vi "Read Waveform.vi"(6 "wait for reply (T)":bool=TRUE, 8 "error in":errorcluster, 10 "Parameters 3":T1, 11 "Module ID":i32=-1) -> (0 "error out":errorcluster, 1 "timed out?":bool)   [LabVIEW 2020, in "Osciloscope Tektronix.lvlib"]
doc: "_____\nCreated using DQMH Event Scripter 6.0.0.122."
uses:
  Osciloscope Tektronix.lvlib
  Read Waveform Argument--cluster.ctl
  Read Waveform (Reply Payload)--cluster.ctl
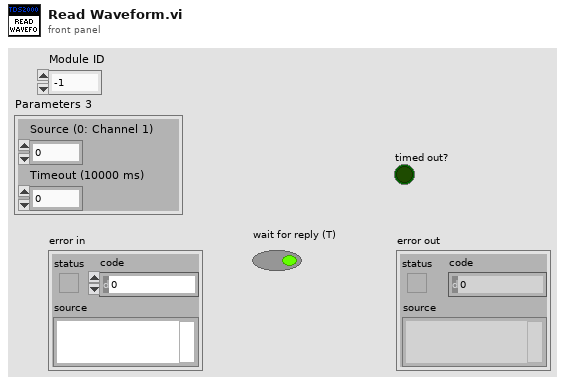
[diagram p1: front panel]
types:
  T1 = cluster{"Source (0: Channel 1)":u16, "Timeout (10000 ms)":u32}
  T2 = typedef "Osciloscope Tektronix.lvlib/Read Waveform Argument--cluster.ctl" = cluster{"Module ID":i32, "Wait Notifier":refnum<notifier>, "wait for reply":bool, "Parameters 3":cluster{"Source (0: Channel 1)":u16, "Timeout (10000 ms)":u32}}
  T3 = typedef "Osciloscope Tektronix.lvlib/Request Events--cluster.ctl" = cluster{"Stop Module":refnum<user-event>, "Show Panel":refnum<user-event>, "Hide Panel":refnum<user-event>, "Show Diagram":refnum<user-event>, "Get Module Execution Status":refnum<user-event>, "SET COM Port":refnum<user-event>, "Initialize Oscilloscope":refnum<user-event>, "Close Oscilloscope":refnum<user-event>, "AutoSetup":refnum<user-event>, "Configure Channel":refnum<user-event>, "Reset":refnum<user-event>, "Read Waveform":refnum<user-event>, "Read Measurement":refnum<user-event>, "Read Measurement 2 channels":refnum<user-event>}
  T4 = typedef "Osciloscope Tektronix.lvlib/Read Waveform (Reply Payload)--cluster.ctl" = cluster{"Read Waveform_error":errorcluster, "Waveform Data":waveform(dbl)}
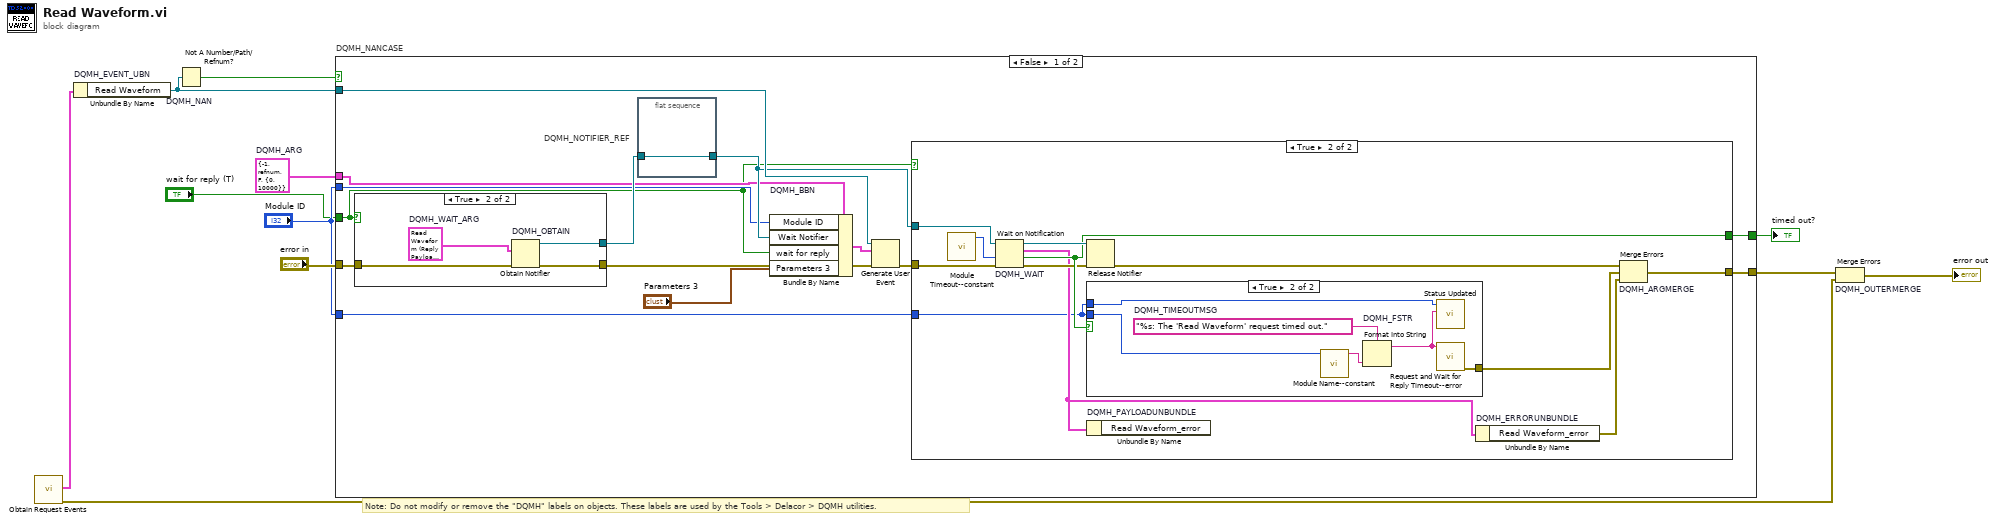
[diagram p0: block diagram]
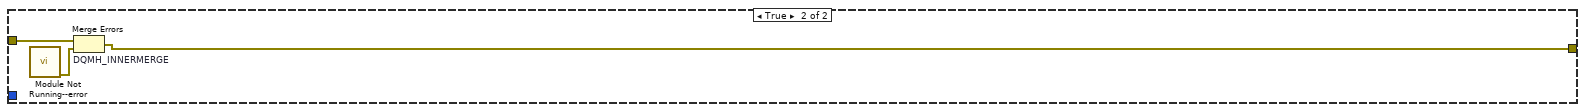
[diagram p5: hidden frame]
diagram:
  w5 = T2 {"Module ID"=-1, "Wait Notifier"=refnum, "wait for reply"=FALSE, "Parameters 3"={"Source (0: Channel 1)"=0, "Timeout (10000 ms)"=10000}}  # DQMH_ARG
  # "Note: Do not modify or remove the \"DQMH\" labels on objects. These labels are used by the Tools > Delacor > DQMH utilities."
  n1 = call "Obtain Request Events.vi"() -> ("error out"=w2:errorcluster, "Osciloscope Tektronix Request Events"=w1:T3)  [unwired: 10 in]
  n2 = Unbundle By Name "DQMH_EVENT_UBN"(w1) -> ("Read Waveform"=w9:refnum<user-event>)
  n3 = Not A Number/Path/Refnum? "DQMH_NAN"(number/path/refnum=w9) -> (NaN/Path/Refnum?=w8:bool)
  n4 = case "DQMH_NANCASE" shown="False" w8 {
    tunnel: "error in" -> [w25 w53]
    tunnel: w9 -> [w23 _]
    tunnel: [w20 w52] -> w6
    tunnel: [w21 _] -> w7
    tunnel: w5 -> [w16 _]
    tunnel: "Module ID" -> [w15 _]
    tunnel: "Module ID" -> [w14 _]
    tunnel: "wait for reply (T)" -> [w13 _]
    frame False {
      n5 = case shown="True" w13 {
        tunnel: w25 -> [w46 w50]
        tunnel: [w46 w49] -> w22
        tunnel: [_ w47] -> w18
        frame False {
        }
        frame True {
          w48 = T4 {"Read Waveform_error"={"status"=FALSE, "code"=0, "source"=""}, "Waveform Data"={"t0"=timestamp(0 s since 1904-01-01), "dt"=1.0, "Y"=[]}}  # DQMH_WAIT_ARG
          n6 = Obtain Notifier "DQMH_OBTAIN"(notification data type=w48, error in (no error)=w50) -> (notifier out=w47:refnum<notifier>, error out=w49:errorcluster)  [unwired: 2 in, 1 out]
        }
      }
      n7 = flat-sequence "DQMH_NOTIFIER_REF" {
        tunnel: w18 -> [w26]
        tunnel: [w26] -> w17
        frame #0 {
        }
      }
      n8 = Bundle By Name "DQMH_BBN"(cluster=w16, "Module ID"=w15, "Wait Notifier"=w17, "wait for reply"=w13, "Parameters 3"="Parameters 3") -> (w19:T2)
      n9 = Generate User Event(user event=w23, event data cluster=w19, error in=w22) -> (error out=w24:errorcluster)  [unwired: 1 in, 1 out]
      n10 = case shown="True" w13 {
        tunnel: w24 -> [w27 w39]
        tunnel: w17 -> [_ w38]
        tunnel: [_ w36] -> w21
        tunnel: [w27 w35] -> w20
        tunnel: w14 -> [_ w28]
        frame False {
        }
        frame True {
          n11 = call "Module Timeout--constant.vi"() -> ("Module Timeout"=w29:i32)  [unwired: 11 in]
          n12 = Wait on Notification "DQMH_WAIT"(notifier=w38, timeout in ms (-1)=w29, error in (no error)=w39) -> (notifier out=w37:refnum<notifier>, notification=w30:T4, timed out?=w36:bool, error out=w34:errorcluster)  [unwired: 1 in]
          n13 = Release Notifier(notifier=w37, error in (no error)=w34) -> (error out=w33:errorcluster)  [unwired: 1 in, 2 out]
          n14 = case shown="True" w36 {
            tunnel: [_ w43] -> w31
            tunnel: w28 -> [_ w41]
            tunnel: w28 -> [_ w40]
            frame False {
            }
            frame True {
              w45 = "%s: The 'Read Waveform' request timed out."  # DQMH_TIMEOUTMSG
              n15 = call "Module Name--constant.vi"("Module ID"=w40) -> ("Module Name"=w42:string)  [unwired: 10 in]
              n16 = Format Into String "DQMH_FSTR"(format string=w45, w42) -> (resulting string=w44:string)  [unwired: 2 in, 1 out]
              n17 = call "Status Updated.vi"("Status"=w44, "Module ID"=w41) -> ()  [unwired: 9 in, 1 out]
              n18 = call "Request and Wait for Reply Timeout--error.vi"("Error Message"=w44) -> ("error out"=w43:errorcluster)  [unwired: 10 in]
            }
          }
          n19 = Unbundle By Name "DQMH_PAYLOADUNBUNDLE"(w30) -> ()  [unwired: 1 out]
          n20 = Unbundle By Name "DQMH_ERRORUNBUNDLE"(w30) -> ("Read Waveform_error"=w32:errorcluster)
          n21 = Merge Errors "DQMH_ARGMERGE"(w33, w31, w32) -> (w35:errorcluster)
        }
      }
    }
    frame True {
      n22 = call "Module Not Running--error.vi"() -> ("error out"=w51:errorcluster)  [unwired: 11 in]
      n23 = Merge Errors "DQMH_INNERMERGE"(w53, w51) -> (w52:errorcluster)
    }
  }
  "timed out?" <- w7
  n24 = Merge Errors "DQMH_OUTERMERGE"(w6, w2) -> (→"error out":errorcluster)
